vi "CSM - Convert HexStr to Data.vi"(2 "HEX String":string, 3 "error in (no error)":errorcluster) -> (7 "Variant":variant, 9 "error out":errorcluster)   [LabVIEW 2020, in "Communicable State Machine.lvlib"]
doc: "Convert hex string arguments back to variant.\n\n<b>Inputs:</b>\n - <b>HEX String</b>: Hex String, which contains no invisible string following CSM's rule\n\n<b>Outputs:</b>\n - <b>Variant</b>: Complex data in variant format.\n - <b>error out</b>: Error output"
uses:
  Communicable State Machine.lvlib
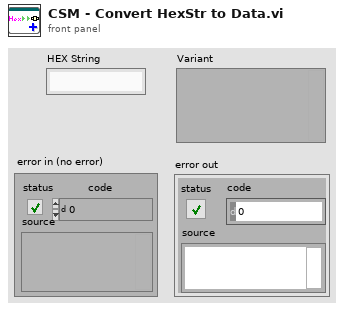
[diagram p1: front panel]
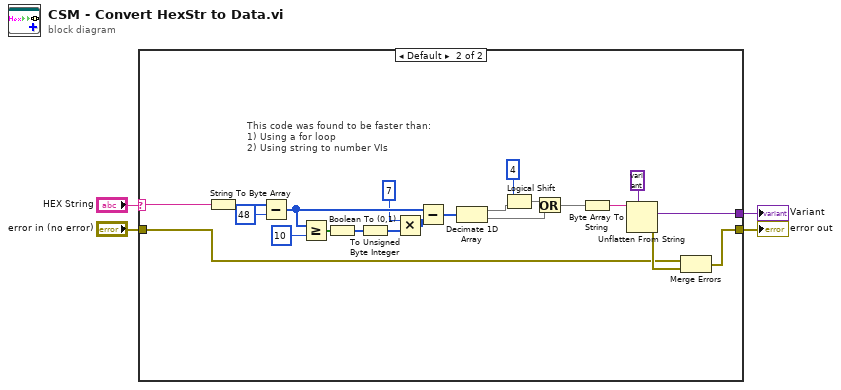
[diagram p0: block diagram]
diagram:
  n1 = case shown="Default" "HEX String" {
    selector: "HEX String" -> [_ w10]
    tunnel: [_ w26] -> w4
    tunnel: [w5 w7] -> w2
    tunnel: "error in (no error)" -> [w5 w6]
    frame "" {
    }
    frame Default {
      # "This code was found to be faster than:\n1) Using a for loop\n2) Using string to number VIs"
      n2 = String To Byte Array(string=w10) -> (unsigned byte array=w11:u8[])
      n3 = Subtract(x=w11, y=u8 48) -> (x-y=w22:u8[])
      n4 = Greater Or Equal?(x=w22, y=u8 10) -> (x >= y?=w19:bool[])
      n5 = Boolean To (0,1)(Boolean=w19) -> (0, 1=w17:i16[])
      n6 = To Unsigned Byte Integer(number=w17) -> (unsigned 8bit integer=w20:u8[])
      n7 = Multiply(x=u8 7, y=w20) -> (x*y=w21:u8[])
      n8 = Subtract(x=w22, y=w21) -> (x-y=w13:u8[])
      n9 = Decimate 1D Array(w13) -> (w14:u8[], w12:u8[])
      n10 = Logical Shift(y=i8 4, x=w14) -> (x << y=w23:u8[])
      n11 = Or(x=w23, y=w12) -> (x .or. y?=w9:u8[])
      n12 = Byte Array To String(unsigned byte array=w9) -> (string=w25:string)
      n13 = Unflatten From String(type=variant, binary string=w25) -> (value=w26:variant, error out=w8:errorcluster)  [unwired: 3 in, 1 out]
      n14 = Merge Errors(w6, w8) -> (w7:errorcluster)
    }
  }
  "Variant" <- w4
  "error out" <- w2
